vi "Notify All Objects.vi"(8 "error in (no error)":errorcluster, 11 "StorageService in":refnum<class "StorageService.lvclass">) -> (0 "error out":errorcluster, 3 "StorageService out":refnum<class "StorageService.lvclass">)   [LabVIEW 2014, in "StorageService.lvclass"]
uses:
  StorageService.lvclass
  <vilib>/ActorFramework/Actor/Actor.lvclass/Actor.ctl
  <vilib>/ActorFramework/Message Enqueuer/Message Enqueuer.lvclass/Message Enqueuer.ctl
  StorageService.lvclass/StorageService.ctl
  StorageService Messages/Store Data Msg/Store Data Msg.lvclass
  <vilib>/ActorFramework/Message Enqueuer/Init from Existing Queue.vi
  <vilib>/ActorFramework/Message Enqueuer/Message Enqueuer.lvclass
  <vilib>/ActorFramework/Actor/Actor.lvclass
  Model/ReplayData Msg/ReplayData Msg.lvclass
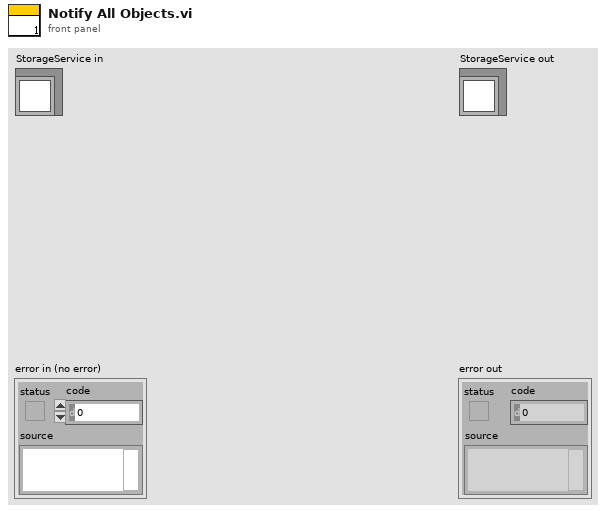
[diagram p1: front panel]
types:
  T1 = typedef "StorageService.lvclass/RegisteredObject.ctl" = cluster{"Name":string, "Is Acquired":bool, "Queue":refnum<queue>, "Message To Send":cluster{"Enqueuer":refnum<class "Message Enqueuer.lvclass">, "Message":refnum<class "ReplayData Msg.lvclass">}, "Save Parameters":variant}
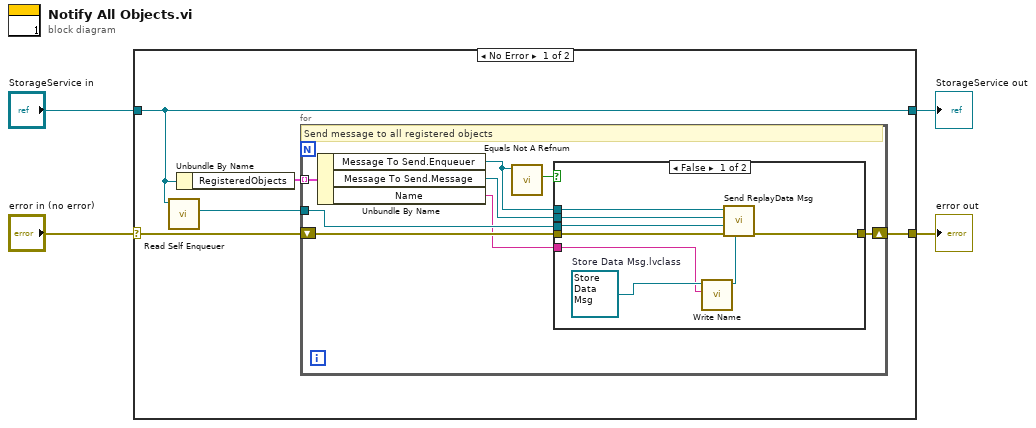
[diagram p0: block diagram]
diagram:
  n1 = case shown="No Error" "error in (no error)" {
    selector: "error in (no error)" -> [w8 w28]
    tunnel: [w7 w28] -> w3
    tunnel: [w6 w27] -> w1
    tunnel: "StorageService in" -> [w6 w27]
    frame No Error {
      n2 = call <vilib>:"Read Self Enqueuer.vi"("Actor"=w6) -> ("Self Enqueuer"=w5:refnum<class "Message Enqueuer.lvclass">)  [unwired: 10 in]
      n3 = Unbundle By Name(w6) -> ("RegisteredObjects"=w9:T1[])
      n4 = for {
        tunnel: w9 -> [w17] mode=indexing
        shift-right: [w12] -> w7
        shift-left: w8 -> [w13]
        tunnel: w5 -> [w11]
        # "Send message to all registered objects"
        n5 = Unbundle By Name(w17) -> ("Message To Send.Enqueuer"=w14:refnum<class "Message Enqueuer.lvclass">, "Message To Send.Message"=w15:refnum<class "ReplayData Msg.lvclass">, "Name"=w10:string)
        n6 = call <vilib>:"Equals Not A Refnum.vi"("Message Enqueuer"=w14) -> ("Not a refnum?"=w16:bool)  [unwired: 10 in]
        n7 = case shown="False" w16 {
          tunnel: w15 -> [w24 _]
          tunnel: w14 -> [w25 _]
          tunnel: w13 -> [w22 w26]
          tunnel: [w21 w26] -> w12
          tunnel: w11 -> [w23 _]
          tunnel: w10 -> [w18 _]
          frame False {
            w19 = refnum<class "Store Data Msg.lvclass"> refnum  # Store Data Msg.lvclass
            n8 = call-dynamic "Write Name.vi"("Name"=w18, "Data Msg in"=w19) -> ("Data Msg out"=w20:refnum<class "Store Data Msg.lvclass">)  [unwired: 8 in, 1 out]
            n9 = call "Send ReplayData Msg.vi"("On End Message"=w20, "error in (no error)"=w22, "Caller Enqueuer"=w23, "ReplayData Msg"=w24, "Message Enqueuer"=w25) -> ("error out"=w21:errorcluster)  [unwired: 5 in, 1 out]
          }
          frame True {
          }
        }
      }
    }
    frame Error {
    }
  }
  "error out" <- w3
  "StorageService out" <- w1
